vi "SRV_Create User Exit Event.vi"(8 "error in (no error)":errorcluster) -> (0 "error out":errorcluster, 3 "User Exit Event":refnum<user-event>)   [LabVIEW 2009]
doc: "Wire the output in to a Register For Events node.\n\n\nAuthor: Mike Schultz\n\n\nLogicPD, Inc\nwww.logicpd.com"
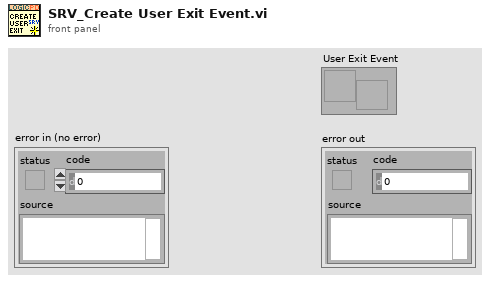
[diagram p1: front panel]
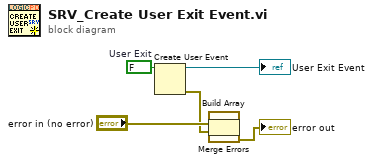
[diagram p0: block diagram]
diagram:
  w5 = FALSE  # User Exit
  n1 = Create User Event(user event datatype=w5) -> (user event=→"User Exit Event":refnum<user-event>, error out=w3:errorcluster)  [unwired: 1 in]
  n2 = Build Array("error in (no error)", w3) -> (w1:errorcluster[])
  n3 = call <vilib>:"Merge Errors.vi"("error array in"=w1) -> ("error out"=→"error out":errorcluster)  [unwired: 6 in]
